vi "Launch Visualization Communication.vi"(8 "error in (no error)":errorcluster, 11 "Master Controller in":refnum<class "Master Controller.lvclass">) -> (0 "error out":errorcluster, 3 "Master Controller out":refnum<class "Master Controller.lvclass">)   [LabVIEW 2015, in "Master Controller Core.lvlib" / "Master Controller.lvclass"]
uses:
  Master Controller.lvclass
  Communications/SCADA Communcations Actor/SCADA Communications/SCADA Communications.lvclass
  Communications/SCADA Communcations Actor/SCADA Communications Messages/EMS Message Msg/EMS Message Msg.lvclass
  Master Controller Messages/Read EMS Message Msg/Read EMS Message Msg.lvclass
  Communications/TCPIP Communications Framework/TCPIP Communications/Controls/Mode Select.ctl
  Communications/SCADA Communcations Actor/SCADA Communications/SCADA Communications.lvclass/SCADA Communications.ctl
  Master Controller.lvclass/Master Controller.ctl
  Communications/TCPIP Communications Framework/TCPIP Communications/TCPIP Communications.lvclass/TCPIP Communications.ctl
  <vilib>/ActorFramework/Actor/Actor.lvclass
  Communications/TCPIP Communications Framework/TCPIP Communications/TCPIP Communications.lvclass
  Utilities/Status Messaging.llb/Status Messaging.lvlib
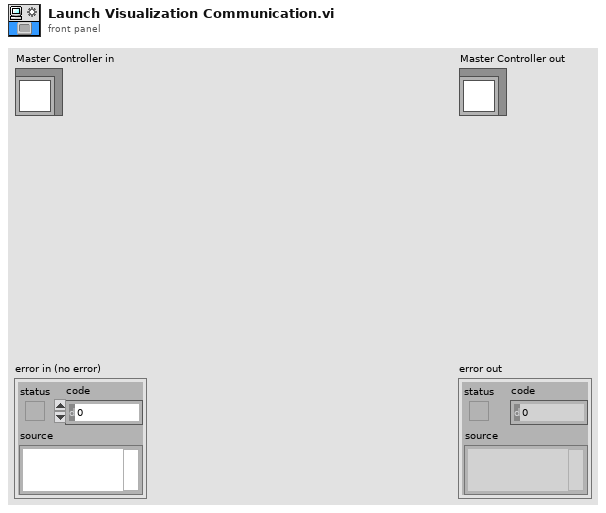
[diagram p1: front panel]
types:
  T1 = typedef "TCPIP Communications Framework.lvlib/TCPIP Communications.lvclass/Mode Select.ctl" = enum16{"Tx/Rx", "Tx", "Rx"}
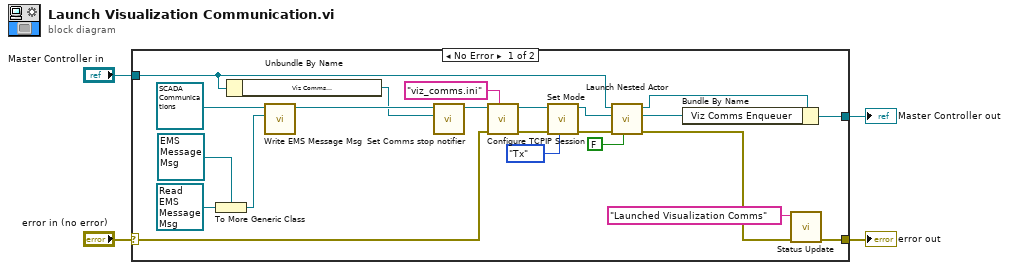
[diagram p0: block diagram]
diagram:
  n1 = case shown="No Error" "error in (no error)" {
    selector: "error in (no error)" -> [w26 w28]
    tunnel: [w11 w28] -> w3
    tunnel: [w24 w27] -> w1
    tunnel: "Master Controller in" -> [w7 w27]
    frame No Error {
      n2 = To More Generic Class(target class=refnum<class "EMS Message Msg.lvclass"> refnum ("SCADA Communcations Actor.lvlib:EMS Message Msg.lvclass"), reference=refnum<class "Read EMS Message Msg.lvclass"> refnum ("Master Controller Core.lvlib:Read EMS Message Msg.lvclass")) -> (generic class reference=w19:refnum<class "EMS Message Msg.lvclass">)
      n3 = Unbundle By Name(w7) -> ("Viz Comms\nstop"=w6:refnum<notifier>)
      n4 = call "Write EMS Message Msg.vi"("EMS Message Msg"=w19, "SCADA Communications in"=refnum<class "SCADA Communications.lvclass"> refnum ("SCADA Communcations Actor.lvlib:SCADA Communications.lvclass")) -> ("SCADA Communications out"=w9:refnum<class "SCADA Communications.lvclass">)  [unwired: 9 in]
      n5 = call "Set Comms stop notifier.vi"("Comms stop"=w6, "SCADA Communications in"=w9) -> ("SCADA Communications out"=w8:refnum<class "SCADA Communications.lvclass">)  [unwired: 9 in]
      n6 = call "Configure TCPIP Session.vi"("config file name"="viz_comms.ini", "error in (no error)"=w26, "TCPIP Communications in"=w8) -> ("error out"=w17:errorcluster, "TCPIP Communications out"=w16:refnum<class "SCADA Communications.lvclass">)  [unwired: 7 in]
      n7 = call "Set Mode.vi"("Mode"=Mode_Select."Tx", "error in (no error)"=w17, "TCPIP Communications in"=w16) -> ("error out"=w15:errorcluster, "TCPIP Communications out"=w14:refnum<class "SCADA Communications.lvclass">)  [unwired: 7 in]
      n8 = call <vilib>:"Launch Nested Actor.vi"("Open Actor Core front panel? (F)"=FALSE, "error in (no error)"=w15, "Nested Actor"=w14, "Caller Actor in"=w7) -> ("error out"=w12:errorcluster, "Nested Actor's Enqueuer"=w23:refnum<class "Message Enqueuer.lvclass">, "Caller Actor out"=w25:refnum<class "Master Controller.lvclass">)  [unwired: 5 in]
      n9 = Bundle By Name(cluster=w25, "Viz Comms Enqueuer"=w23) -> (w24:refnum<class "Master Controller.lvclass">)
      n10 = call "Status Update.vi"("error in (no error)"=w12, "Status Update"="Launched Visualization Comms") -> ("error out"=w11:errorcluster)  [unwired: 8 in, 1 out]
    }
    frame Error {
    }
  }
  "error out" <- w3
  "Master Controller out" <- w1
